vi "Stop FPGA Acquisition.vi"(8 "Error In":errorcluster) -> (0 "Error Out":errorcluster, 3 "FPGA Ref":T1)   [LabVIEW 2017]
doc: "Stops the acquisition."
uses:
  RIG-SPECIFIC FILES/FPGA Refs/FPGA Ref.ctl
  Typedefs/HW config states enum.ctl
  <vilib>/Utility/error.llb/Error Cluster From Error Code.vi
  <vilib>/rvi/interface/nirviMethod/nirviMethod.xnode
  <vilib>/rvi/errors/niLvFpgaMergeErrorWithErrorCode.vi
  <vilib>/FPGAPlugInAG/Dynamic/niLvFpga_StopFifo_Dynamic.vi
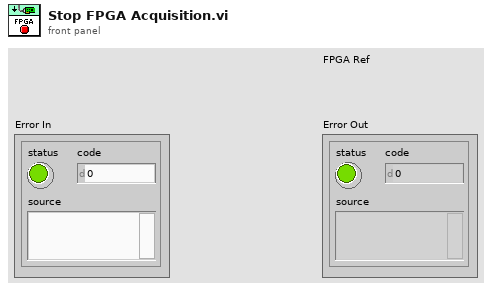
[diagram p1: front panel]
types:
  T1 = typedef "FPGA Ref.ctl" = refnum<k20>
  T2 = typedef "HW config states enum.ctl" = enum16{"Load from file", "Save to file", "Write all", "Read all", "Write XY stage settings", "Write DAQ FPGA settings", "Write Control FPGA settings", "Write Phys Channels", "Write System Config", "Write HW Config", "Save System Config", "Save HW Config", "Clear", "Compare from file"}
  T3 = typedef "Hardware Configuration settings.ctl" = cluster{"Dev. PC":bool, "Swap XY on stage":bool, "No of AOD":u8, "MC Supported":bool, "Axial MC":bool, "Computer MAC address":string, "Externalise Triggers":bool, "Trigger HW config":T4, "DAQmx Chan":T5, "XY stage available":bool, "XY Stage":T6, "Z stage available":bool, "Z Stage config cluster":T7, "Encoder available":bool, "Encoder":T8, "VidRec available":bool, "Cam VidRec":T9, "Laser Power Control HW config":T10, "Laser 1 available":bool, "Laser 1 config cluster":T11, "Prechirper 1 available":bool, "Prechirper 1 config cluster":T12, "Control system.FPGA available?":bool, "Control Sys. HW config":T13, "DAQ FPGA HW Config":T14}
  T4 = typedef "Triggers HW config.ctl" = cluster{"Available Device List":i32, "Device Address":string}
  T5 = typedef "DAQmx physical channels cluster.ctl" = cluster{"Pockels AO":tag, "Hard shutter AO":tag, "PMT AOs":tag, "Galvo AOs":tag, "Power meter AI":tag}
  T6 = typedef "XY Stage config cluster.ctl" = cluster{"COM port":refnum<visa-resource-name>, "Baudrate":i32, "Type":string}
  T7 = typedef "Z Stage config cluster.ctl" = cluster{"COM port":refnum<visa-resource-name>, "Baudrate":i32, "Type":string}
  T8 = typedef "Encoder config cluster.ctl" = cluster{"IP address":string, "Port":u16, "Wheel radius (cm)":dbl, "Encoder Trigger":tag}
  T9 = typedef "Cam VidRec HW config setup cluster.ctl" = cluster{"DO flag-Video record":tag, "DO flag-Trial start":tag}
  T10 = typedef "Laser Power Control HW config.ctl" = cluster{"Laser Power Control":string, "Laser Power Modulation Control":enum16{"NI", "FPGA"}}
  T11 = typedef "Laser 1 config cluster.ctl" = cluster{"COM port":refnum<visa-resource-name>, "Baud Rate":i32, "Type":string}
  T12 = typedef "PreChirper 1 config cluster.ctl" = cluster{"Type":string, "Baud Rate":i32, "COM port":refnum<visa-resource-name>}
  T13 = typedef "Control Sys HW config cluster.ctl" = cluster{"Control system.FPGA Type":enum16{"Virtex 5", "Virtex 7"}, "Control system.Network adapter name":string, "Control system.MAC address":string, "Control system.Ethernet Port":u32, "Control system.Ethernet Port Opened":bool}
  T14 = typedef "DAQ FPGA HW config cluster.ctl" = cluster{"FGPA Ref":T1, "Target":T15, "input card type":T16}
  T15 = typedef "nirio_resource_hc.ctl" = tag
  T16 = typedef "FPGA input type AC-DC.ctl" = enum16{"AC Card", "DC Card"}
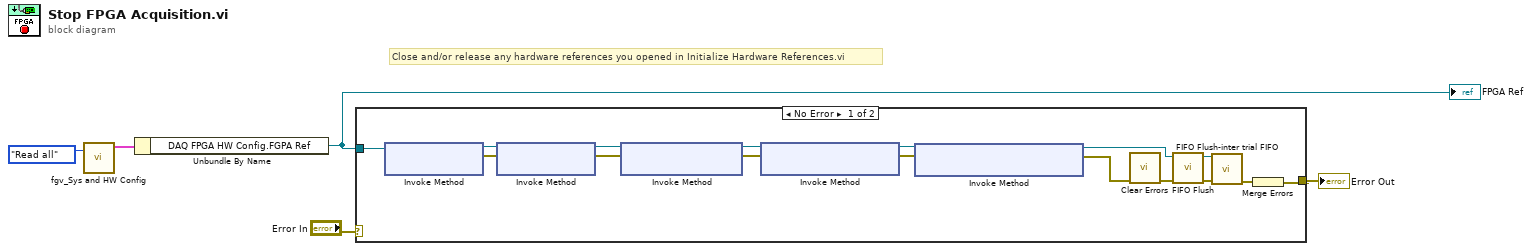
[diagram p0: block diagram]
diagram:
  # "Close and/or release any hardware references you opened in Initialize Hardware References.vi"
  n1 = call "fgv_Sys and HW Config.vi"("Function"=HW_config_states_enum."Read all") -> ("Hardware Configuration OUT"=w1:T3)  [unwired: 8 in, 2 out]
  n2 = Unbundle By Name(w1) -> ("DAQ FPGA HW Config.FGPA Ref"=w2:T1)
  "FPGA Ref" <- w2
  n3 = case shown="No Error" "Error In" {
    selector: "Error In" -> [_ w22]
    tunnel: [w21 w22] -> w4
    tunnel: w2 -> [w17 _]
    frame No Error {
      n4 = xnode "Invoke Method"("FPGA VI Reference In"=w17) -> ("FPGA VI Reference Out"=w20:T1, "error out"=w19:errorcluster)  [unwired: 1 in]
      n5 = xnode "Invoke Method"("FPGA VI Reference In"=w20, "error in"=w19) -> ("FPGA VI Reference Out"=w16:T1, "error out"=w15:errorcluster)
      n6 = xnode "Invoke Method"("FPGA VI Reference In"=w16, "error in"=w15) -> ("FPGA VI Reference Out"=w14:T1, "error out"=w13:errorcluster)
      n7 = xnode "Invoke Method"("FPGA VI Reference In"=w14, "error in"=w13) -> ("FPGA VI Reference Out"=w12:T1, "error out"=w11:errorcluster)
      n8 = xnode "Invoke Method"("FPGA VI Reference In"=w12, "error in"=w11) -> ("FPGA VI Reference Out"=w10:T1, "error out"=w9:errorcluster)
      n9 = call <vilib>:"Clear Errors.vi"("error in (no error)"=w9) -> ("error out"=w18:errorcluster)  [unwired: 5 in, 1 out]
      n10 = call "FIFO Flush.vi"("Error In"=w18, "FPGA VI Ref"=w10) -> ("Error Out"=w8:errorcluster, "FPGA VI Reference Out"=w7:T1)  [unwired: 7 in, 1 out]
      n11 = call "FIFO Flush-inter trial FIFO.vi"("error in"=w8, "FPGA VI Ref"=w7) -> ("error out"=w6:errorcluster)  [unwired: 8 in, 1 out]
      n12 = Merge Errors(w6) -> (w21:errorcluster)
    }
    frame Error {
    }
  }
  "Error Out" <- w4
